vi "Load Reference.vi"(8 "error in (no error)":errorcluster, 10 "Reference":refnum<vi>, 11 "MulticolumnListboxSelection in":refnum<class "MulticolumnListboxSelection.lvclass">) -> (0 "error out":errorcluster, 3 "MulticolumnListboxSelection out":refnum<class "MulticolumnListboxSelection.lvclass">)   [LabVIEW 2015, in "MulticolumnListboxSelection.lvclass"]
doc: "The <b>Load Reference VI</b> is a dynamic dispatch VI that must be overwritten in every QControl Class and must <b>Call Parent Method</b>. This recursively loads the reference of the control to the data space for the Control Class up the inheritance hierarchy (class hierarchy). These references must be loaded in this way to use all of the built-in properties.\n\nThe reference input is the reference type needed for the control but is coerced to Generic. It should be cast back to the correct type before bundling into the class private data. The pre-casted \"Generic\" reference is wired as input to the <b>Call Parent Method</b>.\n<b> </b> <b> </b>\n©2016 Q Software Innovations, LLC (QSI)\nwritten by Quentin Alldredge\nproduced in LabVIEW 2015\n\nsupport@qsoftwareinnovations.com\nwww.qsoftwareinnovations.com\n\nAll rights reserved.\n\nRedistribution and use in source and binary forms, with or without modification, are permitted provided that the following conditions are met:\n\n * Redistributions of source code must retain the above copyright notice, this list of conditions and the following disclaimer.\n * Redistributions in binary form must reproduce the above copyright notice, this list of conditions and the following disclaimer in the documentation and/or other materials provided with the distribution.\n * Neither the name of Q Software Innovations, LLC. nor the names of its contributors may be used to endorse or promote products derived from this software without specific prior written permission.\n\nTHIS SOFTWARE IS PROVIDED BY THE COPYRIGHT HOLDERS AND CONTRIBUTORS \"AS IS\" AND ANY EXPRESS OR IMPLIED WARRANTIES, INCLUDING, BUT NOT LIMITED TO, THE IMPLIED WARRANTIES OF MERCHANTABILITY AND FITNESS FOR A PARTICULAR PURPOSE ARE DISCLAIMED. IN NO EVENT SHALL THE COPYRIGHT OWNER OR CONTRIBUTORS BE LIABLE FOR ANY DIRECT, INDIRECT, INCIDENTAL, SPECIAL, EXEMPLARY, OR CONSEQUENTIAL DAMAGES (INCLUDING, BUT NOT LIMITED TO, PROCUREMENT OF SUBSTITUTE GOODS OR SERVICES; LOSS OF USE, DATA, OR PROFITS; OR BUSINESS INTERRUPTION) HOWEVER CAUSED AND ON ANY THEORY OF LIABILITY, WHETHER IN CONTRACT, STRICT LIABILITY, OR TORT (INCLUDING NEGLIGENCE OR OTHERWISE) ARISING IN ANY WAY OUT OF THE USE OF THIS SOFTWARE, EVEN IF ADVISED OF THE POSSIBILITY OF SUCH DAMAGE."
uses:
  MulticolumnListboxSelection.lvclass
  MulticolumnListboxSelection.lvclass/MulticolumnListboxSelection.ctl
  MulticolumnListbox/MulticolumnListbox.lvclass
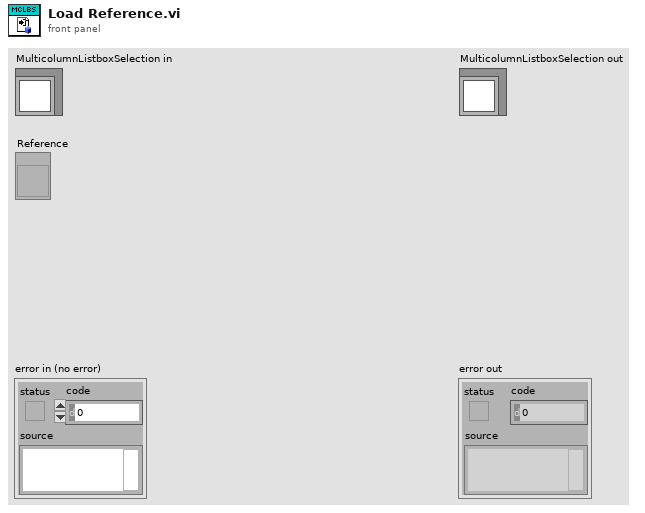
[diagram p1: front panel]
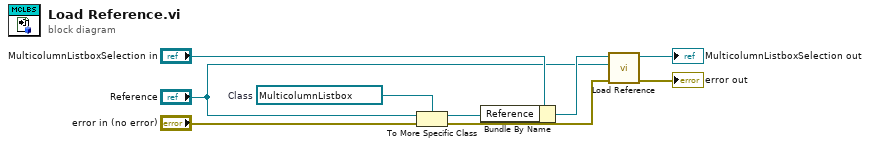
[diagram p0: block diagram]
diagram:
  w4 = refnum<vi> refnum  # Class
  n1 = To More Specific Class(target class=w4, reference="Reference", error in="error in (no error)") -> (specific class reference=w1:refnum<vi>, error out=w2:errorcluster)
  n2 = Bundle By Name(cluster="MulticolumnListboxSelection in", "Reference"=w1) -> (w7:refnum<class "MulticolumnListboxSelection.lvclass">)
  n3 = call-parent "Load Reference.vi"("error in (no error)"=w2, "Reference"="Reference", "MulticolumnListbox in"=w7) -> ("error out"=→"error out":errorcluster, "MulticolumnListbox out"=→"MulticolumnListboxSelection out":refnum<class "MulticolumnListboxSelection.lvclass">)  [unwired: 7 in]
